vi "test harness_FXP_Matrix_Vector_mult_loop_32bit.vi"(8 "error in (no error)":errorcluster, 11 "TestCase in":refnum<class "FXP_observer_TestCase.lvclass">) -> (0 "error out":errorcluster, 3 "TestCase out":refnum<class "FXP_observer_TestCase.lvclass">)   [LabVIEW 2017, in "FXP_observer_TestCase.lvclass"]
uses:
  FXP_observer_TestCase.lvclass
  <vilib>/rvi/DesktopExecutionNode/DesktopExecutionNode.xnode
  <vilib>/rvi/DesktopExecutionNode/Execution/niFpgaDEN_Execute.vi
panel:
  out "xk_1_1_mem":fxp<+/-,32,5>[](array[numeric])
  out "xk_plus1":fxp<+/-,32,7>[](array[numeric])
  out "A*xk (expected)":fxp<+/-,64,12>[](array[numeric])
  in  "Az_mat":fxp<+/-,32,5>[][](array[numeric])=[[1.0, 2.0, 3.0, 4.0], [1.0, 2.0, 2.0, 3.0], [-4.0, -1.0, -3.0, -2.0], [1.0, 5.0, 1.0, 2.0]]
  in  "x_k":fxp<+/-,32,5>[](array[numeric])=[0.10000000149011612, 0.20000000298023224, 0.29999999701976776, 0.3999999985098839, 0.0, 0.0, 0.0, 0.0, 0.0, 0.0, 0.0, 0.0, 0.0, 0.0, 0.0, 0.0, 0.0, 0.0, 0.0, 0.0, 0.0, 0.0, 0.0, 0.0, 0.0, 0.0, 0.0, 0.0, 0.0, 0.0, 0.0, 0.0, 0.0, 0.0, 0.0, 0.0, 0.0, 0.0, 0.0, 0.0, 0.0, 0.0, 0.0, 0.0, 0.0, 0.0, 0.0, 0.0, 0.0, 0.0]
  in  "NS":u8=4
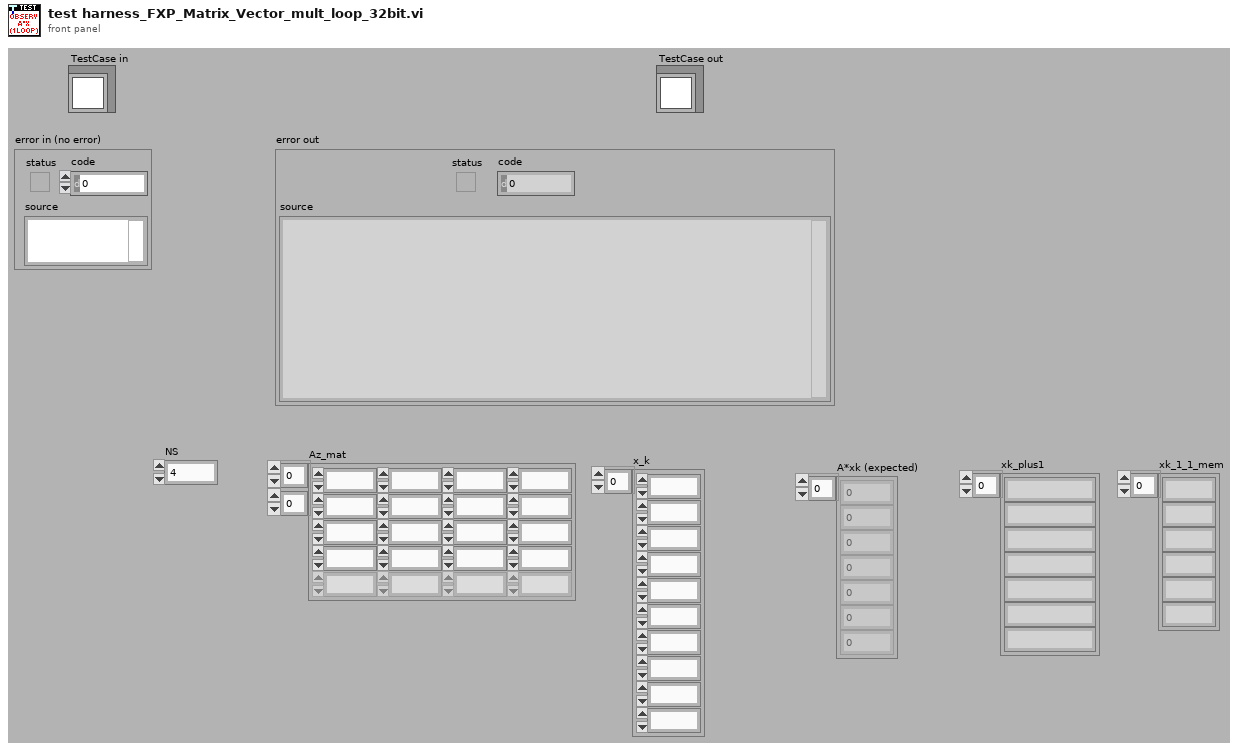
[diagram p1: front panel]
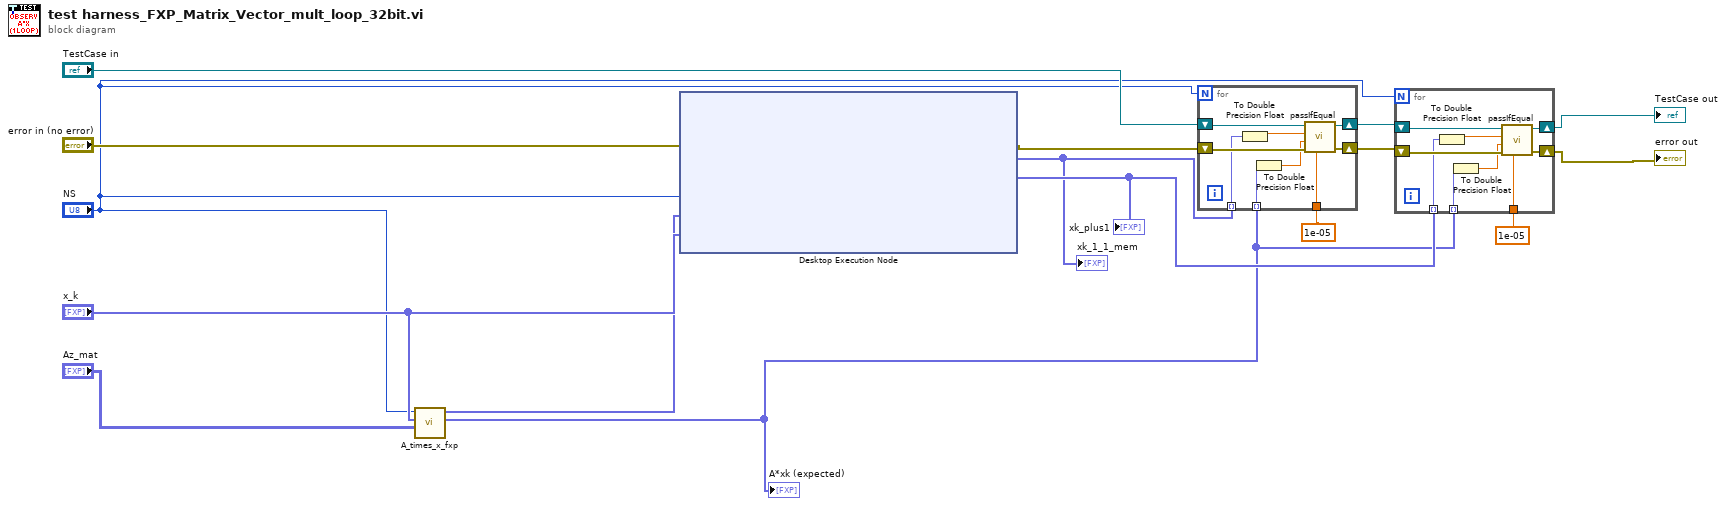
[diagram p0: block diagram]
diagram:
  n1 = call "A_times_x_fxp.vi"("Az_mat in"="Az_mat", "x_k"="x_k", 11:"NS") -> ("A*x"=w3:fxp<+/-,64,12>[], "Az_vec out"=w4:fxp<+/-,32,5>[])  [unwired: 7 in]
  "A*xk (expected)" <- w3
  n2 = xnode "Desktop Execution Node"("Error In"="error in (no error)", "NS + 1"="NS", "Az_col"=w4, "x_k"="x_k") -> ("Error Out"=w9:errorcluster, "xk_1_0_mem"=w1:fxp<+/-,32,6>[], "xk_plus1"=w7:fxp<+/-,32,7>[])
  "xk_plus1" <- w7
  "xk_1_1_mem" <- w1
  n3 = for {
    N: "NS" -> [_]
    shift-right: [w25] -> w12
    shift-left: "TestCase in" -> [w22]
    shift-right: [w24] -> w11
    shift-left: w9 -> [w23]
    tunnel: w3 -> [w21] mode=indexing
    tunnel: 1e-05 ("del u_x") -> [w18]
    tunnel: w1 -> [w17] mode=indexing
    n4 = To Double Precision Float(number=w17) -> (double precision float=w19:dbl)
    n5 = To Double Precision Float(number=w21) -> (double precision float=w20:dbl)
    n6 = call-dynamic "passIfEqual.vi"("delta (optional)"=w18, "error in (no error)"=w23, "y"=w20, "x"=w19, "TestCase in"=w22) -> ("error out"=w24:errorcluster, "TestCase out"=w25:refnum<class "FXP_observer_TestCase.lvclass">)  [unwired: 5 in]
  }
  n7 = for {
    N: "NS" -> [_]
    shift-right: [w34] -> w14
    shift-left: w12 -> [w31]
    shift-right: [w33] -> w15
    shift-left: w11 -> [w32]
    tunnel: w3 -> [w30] mode=indexing
    tunnel: 1e-05 ("del u_x") -> [w27]
    tunnel: w7 -> [w26] mode=indexing
    n8 = To Double Precision Float(number=w26) -> (double precision float=w28:dbl)
    n9 = To Double Precision Float(number=w30) -> (double precision float=w29:dbl)
    n10 = call-dynamic "passIfEqual.vi"("delta (optional)"=w27, "error in (no error)"=w32, "y"=w29, "x"=w28, "TestCase in"=w31) -> ("error out"=w33:errorcluster, "TestCase out"=w34:refnum<class "FXP_observer_TestCase.lvclass">)  [unwired: 5 in]
  }
  "error out" <- w15
  "TestCase out" <- w14
